vi "arcade left code.vi"() -> ()   [LabVIEW 2012, in "joystick.lvrbt"]
uses:
  joystick.lvrbt
  <vilib>/FTC/FTC Read Controller Packet.vi
  <vilib>/NXT/LegoClasses/BrickReference/BrickReference.lvclass
  <vilib>/NXT/Subs/LVHSConnector.ctl
  <vilib>/NXT/NXTIO Xnodes/NXTIOXNode/NXTIO.xnode
  <vilib>/NXT/NXTIO Xnodes/AddressXNode/NXTIOAddress.xnode
  <vilib>/FTC/FTC Calculate Drive Power - Arcade Left.vi
  <vilib>/NXT/Hardware/Plugins/Tetrix DC Motor/TetrixDCMotorAddress.ctl
  <vilib>/NXT/NXTIO Xnodes/NXTIONodeSubVIs/TETRIX IO Move DC Motors.vi
  <vilib>/NXT/NXTIO Xnodes/NXTIONodeSubVIs/TETRIX IO Check Battery.vi
  <vilib>/NXT/NXTIO Xnodes/NXTIONodeSubVIs/TETRIX IO Stop DC Motors.vi
panel:
  in  "Drive Power":i8=75 min=-100 max=100
  # "This VI was generated based on your configuration in the Remote Control Editor. You may modify the code as needed for your robot. To test this program for an FTC match, return to the Remote Control Editor, select the \"Run Program\" tab, and choose \"FTC Game\"."
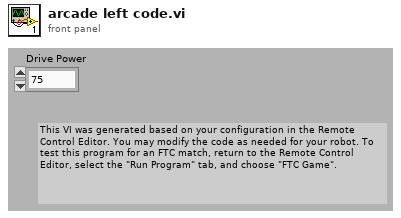
[diagram p1: front panel]
types:
  T1 = typedef "TetrixDCMotorAddress.ctl" = i16
  T2 = cluster{"TetrixDCMotor":T1, "TetrixDCMotor 2":T1}
  T3 = typedef "LVHSConnector.ctl" = refnum<class "BrickReference.lvclass">
  T4 = typedef "FTC ControllerState.ctl" = cluster{"Left X":i8, "Left Y":i8, "Right X":i8, "Right Y":i8, "Button Encoding 9-12":u8, "Button Encoding 1-8":u8, "POV":T5}
  T5 = typedef "FTC POVState.ctl" = i8
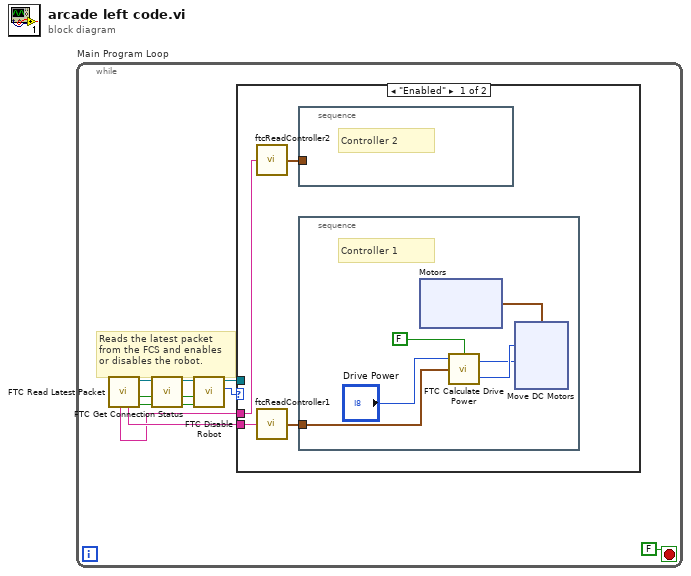
[diagram p0: block diagram]
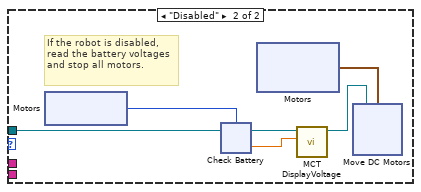
[diagram p2: hidden frame]
diagram:
  n1 = while "Main Program Loop" {
    stop <- FALSE stop-if-true
    # "Reads the latest packet\nfrom the FCS and enables\nor disables the robot."
    n2 = call <vilib>:"FTC Read Latest Packet.vi"() -> ("Packet Received?"=w8:bool, "Stopped?"=w5:bool, "NXT"=w7:T3, "Controller 1"=w10:string, "Controller 2"=w9:string)  [unwired: 6 in, 1 out]
    n3 = call <vilib>:"FTC Get Connection Status.vi"("Packet Received?"=w8, "Stopped?"=w5, "NXT"=w7) -> ("Online?"=w2:bool, "Stopped?"=w3:bool, "NXT"=w4:T3)  [unwired: 5 in]
    n4 = call <vilib>:"FTC Disable Robot.vi"("Online?"=w2, "Stopped?"=w3, "NXT"=w4) -> ("Enabled?"=w6:enum16{"Disabled", "Enabled"}, "NXT"=w1:T3)  [unwired: 3 in]
    n5 = case "disableCase" shown="\"Enabled\"" w6 {
      tunnel: w10 -> [w15 _]
      tunnel: w9 -> [w14 _]
      tunnel: w1 -> [_ w38]
      frame "Enabled" {
        n6 = call "ftcReadController2"("Packet"=w14) -> ("Controller State"=w12:T4)  [unwired: 4 in]
        n7 = call "ftcReadController1"("Packet"=w15) -> ("Controller State"=w13:T4)  [unwired: 4 in]
        n8 = stacked-sequence "controller2Actions" {
          tunnel: w12 -> [_]
          frame #0 {
            # "Controller 2"
          }
        }
        n9 = stacked-sequence "controller1Actions" {
          tunnel: w13 -> [w21]
          frame #0 {
            # "Controller 1"
            n10 = xnode ("Motors")() -> ("Motor"=w18:cluster{"TetrixDCMotor":T1, "TetrixDCMotor":T1})
            n11 = call-poly <vilib>:"FTC Calculate Drive Power.vi"("Reverse"=FALSE, "Controller State"=w21, "Power Level (50)"="Drive Power") -> ("Right Motor Power"=w17:i8, "Left Motor Power"=w16:i8)  [unwired: 1 in]
            n12 = xnode ("Move DC Motors")("Power/Speed 2"=w16, "Power/Speed 1"=w17, "Motors"=w18) -> ()  [unwired: 1 in, 1 out]
          }
        }
      }
      frame "Disabled" {
        # "If the robot is disabled, read the battery voltages and stop all motors."
        n13 = xnode ("Motors")() -> ("Motor"=w37:T1)
        n14 = xnode ("Check Battery")("Motors"=w37, "NXT"=w38) -> ("Voltage 1"=w36:sgl, "NXT"=w35:T3)
        n15 = xnode "Motors"() -> ("Motor"=w34:cluster{"TetrixDCMotor":T1, "TetrixDCMotor":T1})
        n16 = call <vilib>:"MCT DisplayVoltage.vi"("Motor Voltage"=w36, "NXT"=w35) -> ("NXT"=w33:T3)  [unwired: 9 in]
        n17 = xnode "Move DC Motors"("Motors"=w34, "NXT"=w33) -> ()  [unwired: 1 out]
      }
    }
  }
